vi "Update State.vi"(8 "error in (no error)":errorcluster, 9 "Digital Inputs":T1, 10 "Analog Inputs":T2, 11 "GripsMaster in":refnum<class "GripsMaster.lvclass">) -> (0 "error out":errorcluster, 1 "Digital Outputs":T1, 2 "Analog Outputs":T2, 3 "GripsMaster out":refnum<class "GripsMaster.lvclass">)   [LabVIEW 2011, in "GripsMaster.lvclass"]
uses:
  GripsMaster.lvclass
  Controls/Analog Values.ctl
  Controls/Digital Values.ctl
  GripsMaster.lvclass/GripsMaster.ctl
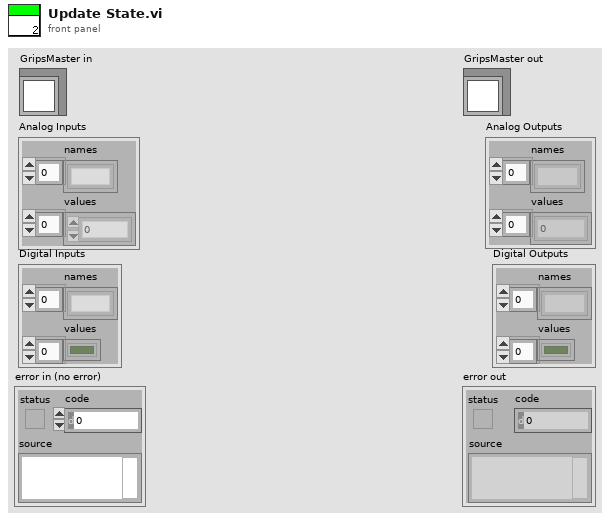
[diagram p1: front panel]
types:
  T1 = typedef "Digital Values.ctl" = cluster{"names":string[], "values":bool[]}
  T2 = typedef "Analog Values.ctl" = cluster{"names":string[], "values":dbl[]}
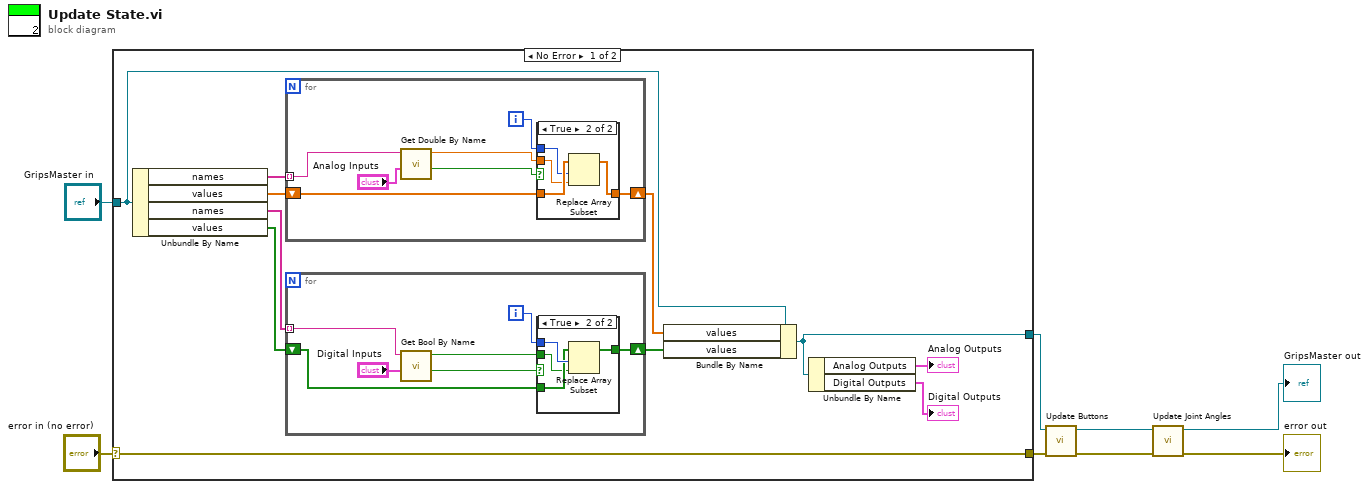
[diagram p0: block diagram]
diagram:
  n1 = case shown="No Error" "error in (no error)" {
    selector: "error in (no error)" -> [w19 w45]
    tunnel: [w19 w45] -> w5
    tunnel: [w16 w44] -> w6
    tunnel: "GripsMaster in" -> [w15 w44]
    frame No Error {
      n2 = Unbundle By Name(w15) -> ("names"=w14:string[], "values"=w13:dbl[], "names"=w11:string[], "values"=w10:bool[])
      n3 = for {
        tunnel: w14 -> [w37] mode=indexing
        shift-right: [w38] -> w12
        shift-left: w13 -> [w36]
        i -> [w35]
        n4 = call "Get Double By Name.vi"("name"=w37, "Analog Values"="Analog Inputs") -> ("result"=w33:dbl, "found?"=w34:bool)  [unwired: 7 in]
        n5 = case shown="True" w34 {
          tunnel: [w39 w43] -> w38
          tunnel: w36 -> [w39 w42]
          tunnel: w35 -> [_ w41]
          tunnel: w33 -> [_ w40]
          frame False {
          }
          frame True {
            n6 = Replace Array Subset(array=w42, new element=w40, index=w41) -> (w43:dbl[])
          }
        }
      }
      n7 = for {
        tunnel: w11 -> [w26] mode=indexing
        shift-right: [w21] -> w9
        shift-left: w10 -> [w23]
        i -> [w22]
        n8 = call "Get Bool By Name.vi"("name"=w26, "Digital Values"="Digital Inputs") -> ("result"=w24:bool, "found?"=w25:bool)  [unwired: 7 in]
        n9 = case shown="True" w25 {
          tunnel: [w27 w31] -> w21
          tunnel: w24 -> [_ w28]
          tunnel: w22 -> [_ w30]
          tunnel: w23 -> [w27 w29]
          frame False {
          }
          frame True {
            n10 = Replace Array Subset(array=w29, new element=w28, index=w30) -> (w31:bool[])
          }
        }
      }
      n11 = Bundle By Name(cluster=w15, "values"=w12, "values"=w9) -> (w16:refnum<class "GripsMaster.lvclass">)
      n12 = Unbundle By Name(w16) -> ("Analog Outputs"=→"Analog Outputs":T2, "Digital Outputs"=→"Digital Outputs":T1)
    }
    frame Error {
    }
  }
  n13 = call "Update Buttons.vi"("error in (no error)"=w5, "GripsMaster in"=w6) -> ("error out"=w3:errorcluster, "GripsMaster out"=w4:refnum<class "GripsMaster.lvclass">)  [unwired: 8 in]
  n14 = call "Update Joint Angles.vi"("error in (no error)"=w3, "GripsMaster in"=w4) -> ("error out"=→"error out":errorcluster, "GripsMaster out"=→"GripsMaster out":refnum<class "GripsMaster.lvclass">)  [unwired: 8 in]
